vi "Command Buffer.vi"(2 "All Robot Commands In":T1, 3 "Startup":bool, 4 "String Parameter":string, 5 "Cmd Parameter 3":dbl, 6 "Cmd Parameter 2":dbl, 7 "Cmd Parameter 1":dbl) -> (0 "All Robot Commands Out":T1, 1 "Completed":bool)   [LabVIEW 2016]
uses:
  Subsystems/All Robot Commands.ctl
  Subsystems/Drive and Climb SS/Drive + Climb Commands 2017.ctl
  Subsystems/Gear Delivery SS/Gear Delivery Commands.ctl
  Subsystems/Conveyor and Shooter SS/Conveyor and Shooter Commands.ctl
  Subsystems/Ball Intake SS/Ball Intake Commands.ctl
  Command Execution State.ctl
  Global Variables/Folder Names.vi
  Global Variables/MotionProfile.vi
  <vilib>/Utility/file.llb/Read Delimited Spreadsheet (DBL).vi
  Global Variables/Refnum Names.vi
panel:
  out "Total Points in File":i32
  # "Sample robot\ncontrol output.\nReplace with \nactual teleop \ncontrol signal \nstructure."
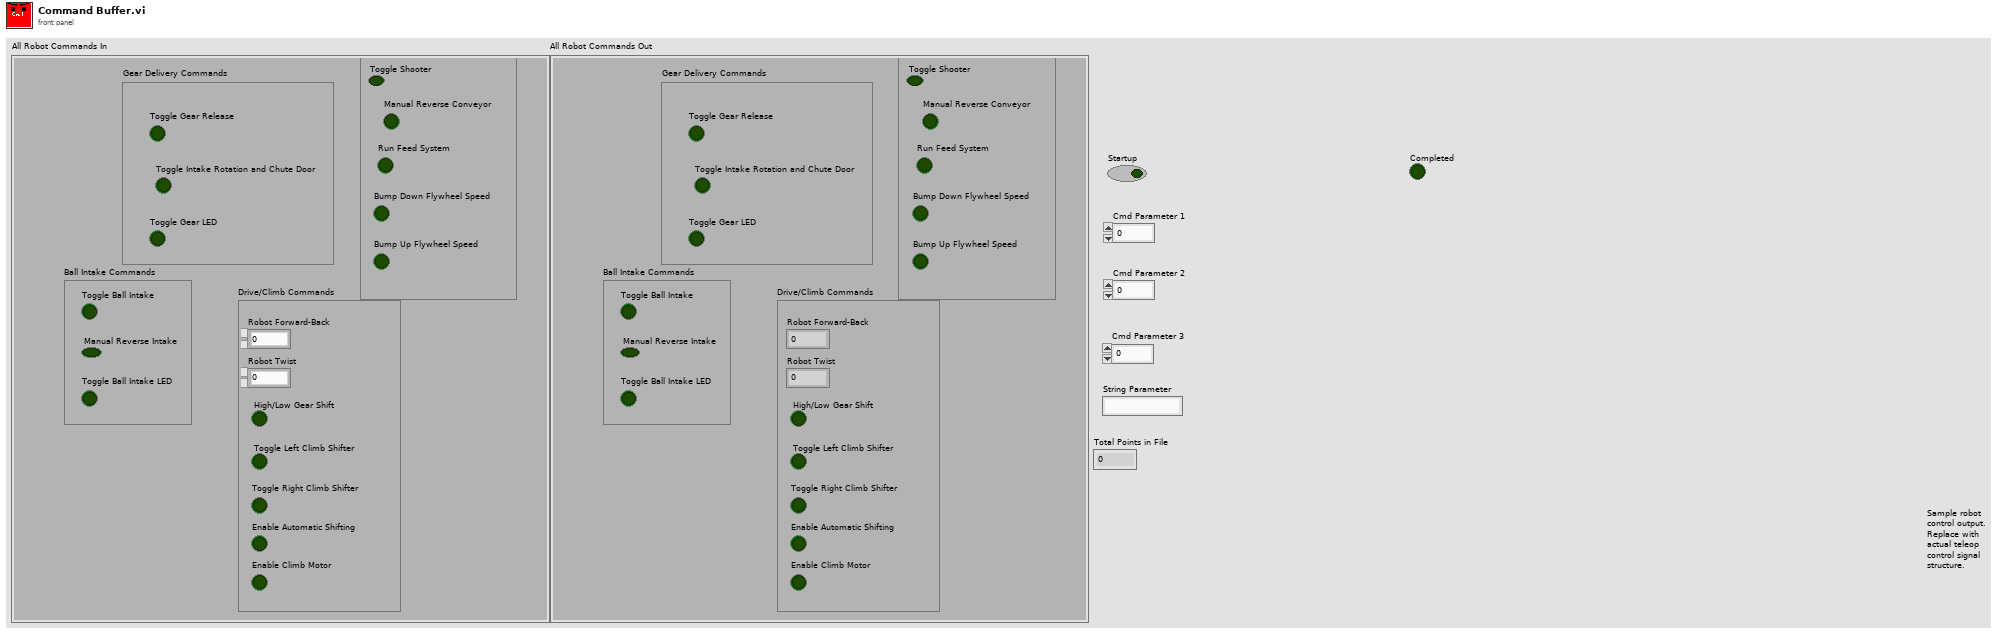
[diagram p1: front panel]
types:
  T1 = typedef "All Robot Commands.ctl" = cluster{"Drive/Climb Commands":T2, "Gear Delivery Commands":T3, "Shooter and Conveyor Commands":T4, "Ball Intake Commands":T5}
  T2 = typedef "Drive + Climb Commands 2017.ctl" = cluster{"Robot Forward-Back":dbl, "Robot Twist":dbl, "High/Low Gear Shift":bool, "Toggle Left Climb Shifter":bool, "Toggle Right Climb Shifter":bool, "Enable Automatic Shifting":bool, "Enable Climb Motor ":bool}
  T3 = typedef "Gear Delivery Commands.ctl" = cluster{"Toggle Gear Release":bool, "Toggle Intake Rotation and Chute Door":bool, "Toggle Gear LED":bool}
  T4 = typedef "Conveyor and Shooter Commands.ctl" = cluster{"Toggle Shooter":bool, "Manual Reverse Conveyor":bool, "Run Feed System":bool, "Bump Down Flywheel Speed":bool, "Bump Up Flywheel Speed":bool}
  T5 = typedef "Ball Intake Commands.ctl" = cluster{"Toggle Ball Intake":bool, "Manual Reverse Intake":bool, "Toggle Ball Intake LED":bool}
  T6 = typedef "Command Execution State.ctl" = enum16{"Initialize", "Execute", "Finish"}
  T7 = typedef "MotionProfile TypeDef.ctl" = cluster{"Left MP Array":dbl[][], "Left MP Index":dbl, "Semaphore":bool, "Right MP Array":dbl[][], "Right MP Index":dbl}
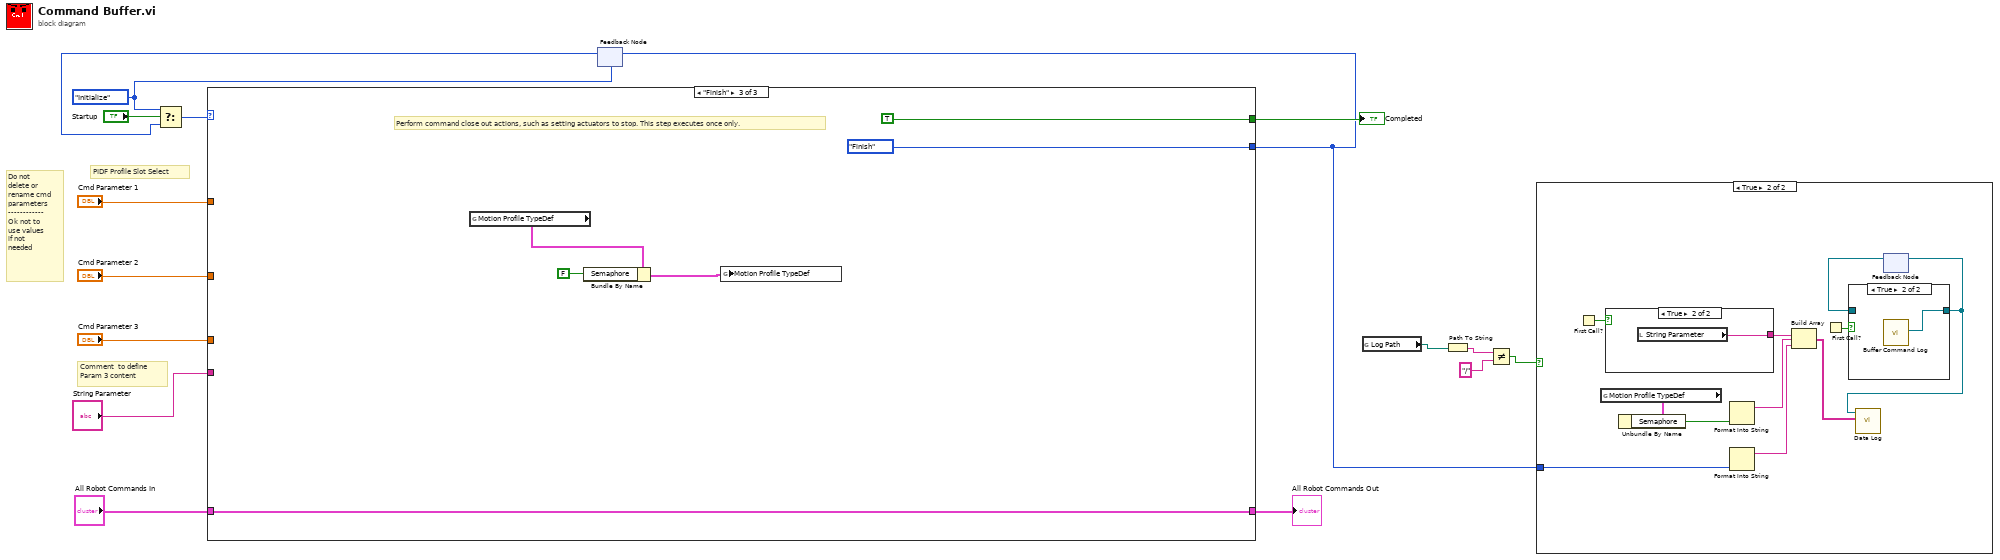
[diagram p0: block diagram]
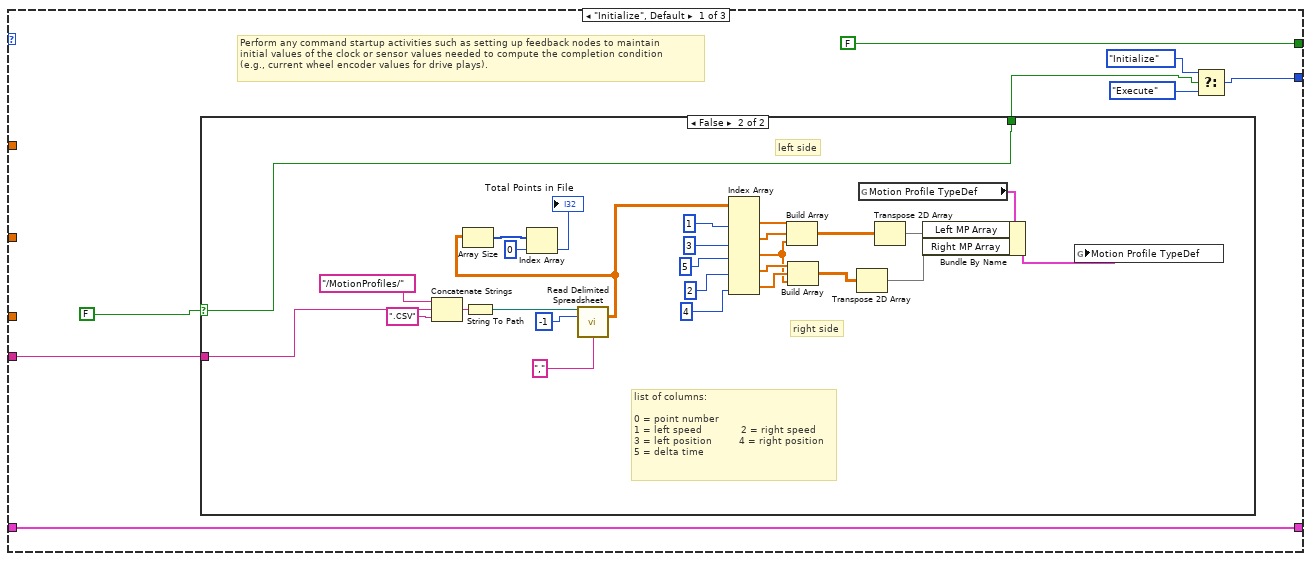
[diagram p5: hidden frame]
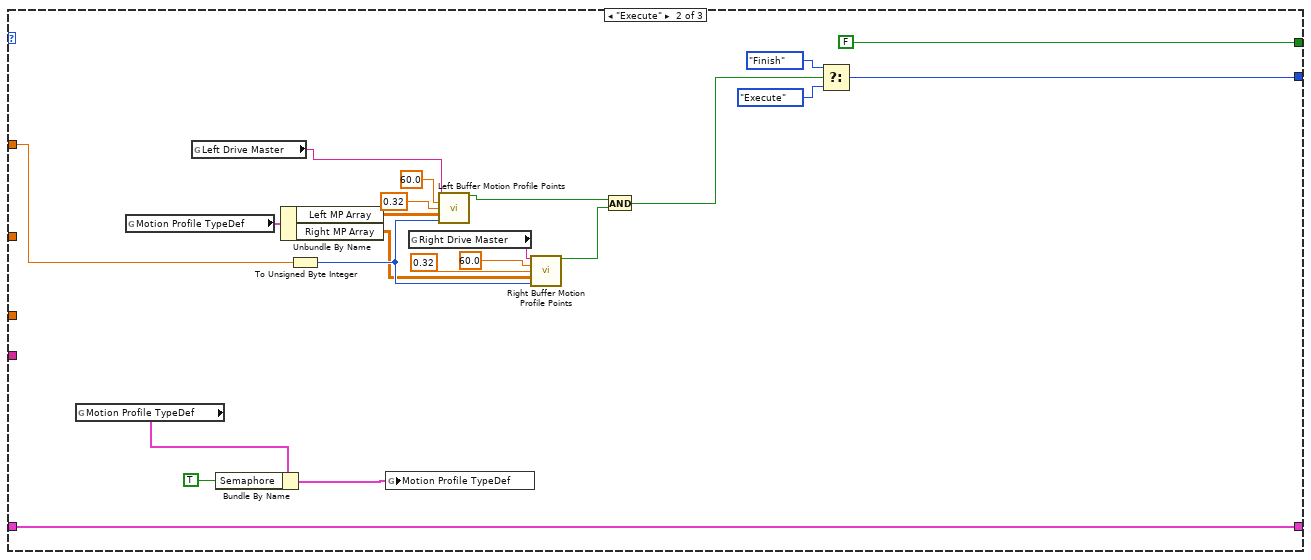
[diagram p7: hidden frame]
diagram:
  w12 = Command_Execution_State."Initialize" ("Play State")
  # "Comment  to define\nParam 3 content"
  # "PIDF Profile Slot Select"
  # "Do not \ndelete or\nrename cmd\nparameters\n------------\nOk not to \nuse values\nif not \nneeded"
  n1 = feedback #1(w12) -> (w13:T6)
  n2 = Select(t=w12, s="Startup", f=w13) -> (s? t:f=w16:T6)
  n3 = case shown="\"Finish\"" w16 {
    tunnel: [FALSE FALSE TRUE] -> w14
    tunnel: [w22 w73 Command_Execution_State."Finish" ("f")] -> w5
    tunnel: "Cmd Parameter 1" -> [_ w68 _]
    tunnel: "Cmd Parameter 2" -> [_ _ _]
    tunnel: "Cmd Parameter 3" -> [_ _ _]
    tunnel: "String Parameter" -> [w23 _ _]
    tunnel: "All Robot Commands In" -> [w18 w54 w76]
    tunnel: [w18 w54 w76] -> w6
    frame "Initialize", Default {
      # "Perform any command startup activities such as setting up feedback nodes to maintain \ninitial values of the clock or sensor values needed to compute the completion condition\n(e.g., current wheel encoder values for drive plays)."
      n4 = case shown="False" FALSE {
        selector: FALSE -> [w25 w27]
        tunnel: w23 -> [_ w50]
        tunnel: [w25 w27] -> w19
        frame True {
        }
        frame False {
          # "list of columns:\n\n0 = point number\n1 = left speed             2 = right speed\n3 = left position         4 = right position\n5 = delta time"
          # "left side"
          # "right side"
          n5 = Concatenate Strings("/MotionProfiles/" ("string"), w50, ".CSV" ("string")) -> (w51:string)
          n6 = String To Path(string=w51) -> (path=w26:path)
          n7 = call-poly <vilib>:"Read Delimited Spreadsheet.vi"("file path (dialog if empty)"=w26, "number of rows (all:-1)"=-1, "delimiter (\\t)"="," ("delimiter (\\t)")) -> ("all rows"=w34:dbl[][])  [unwired: 7 in, 5 out]
          n8 = Array Size(array=w34) -> (size(s)=w33:i32[])
          n9 = Index Array(array=w33, index=0) -> (element=→"Total Points in File":i32)
          n10 = Index Array(array=w34, index (col) #1=1 ("disabled index (col)"), index (col) #2=3 ("disabled index (col)"), index (col) #3=5 ("disabled index (col)"), index (col) #4=2 ("disabled index (col)"), index (col) #5=4 ("disabled index (col)")) -> (element #1=w41:dbl[], element #2=w40:dbl[], element #3=w37:dbl[], element #4=w39:dbl[], element #5=w38:dbl[])  [unwired: 5 in]
          n11 = Build Array(w41, w40, w37) -> (w36:dbl[][])
          n12 = Build Array(w39, w38, w37) -> (w35:dbl[][])
          n13 = Transpose 2D Array(2D array=w35) -> (transposed array=w28:dbl[][])
          n14 = global read "MotionProfile.vi" "Motion Profile TypeDef"() -> (w30:T7)
          n15 = Transpose 2D Array(2D array=w36) -> (transposed array=w29:dbl[][])
          n16 = Bundle By Name(cluster=w30, "Left MP Array"=w29, "Right MP Array"=w28) -> (w31:T7)
          n17 = global write "MotionProfile.vi" "Motion Profile TypeDef"(w31) -> ()
        }
      }
      n18 = Select(t=Command_Execution_State."Initialize" ("Play State"), s=w19, f=Command_Execution_State."Execute" ("Play State")) -> (s? t:f=w22:T6)
    }
    frame "Execute" {
      n19 = global read "MotionProfile.vi" "Motion Profile TypeDef"() -> (w59:T7)
      n20 = global read "MotionProfile.vi" "Motion Profile TypeDef"() -> (w71:T7)
      n21 = global read "Refnum Names.vi" "Left Drive Master"() -> (w56:string)
      n22 = Bundle By Name(cluster=w59, "Semaphore"=TRUE) -> (w57:T7)
      n23 = Unbundle By Name(w71) -> ("Left MP Array"=w70:dbl[][], "Right MP Array"=w63:dbl[][])
      n24 = To Unsigned Byte Integer(number=w68) -> (unsigned 8bit integer=w69:u8)
      n25 = global write "MotionProfile.vi" "Motion Profile TypeDef"(w57) -> ()
      n26 = global read "Refnum Names.vi" "Right Drive Master"() -> (w55:string)
      n27 = call "Left Buffer Motion Profile Points.vi"("Motor Name"=w56, "Time Conversion Factor"=60.0, "Linear Conversion Factor"=0.32, "Motion Profile Array"=w70, "PIDF Profile Slot Select"=w69) -> ("Ready to Execute"=w62:bool)  [unwired: 10 in]
      n28 = call "Right Buffer Motion Profile Points.vi"("Motor Name"=w55, "Time Conversion Factor"=60.0, "Linear Conversion Factor"=0.32, "Motion Profile Array"=w63, "PIDF Profile Slot Select"=w69) -> ("Ready to Execute"=w61:bool)  [unwired: 10 in]
      n29 = And(x=w62, y=w61) -> (x .and. y?=w60:bool)
      n30 = Select(t=Command_Execution_State."Finish" ("Play State"), s=w60, f=Command_Execution_State."Execute") -> (s? t:f=w73:T6)
    }
    frame "Finish" {
      # "Perform command close out actions, such as setting actuators to stop. This step executes once only."
      n31 = global read "MotionProfile.vi" "Motion Profile TypeDef"() -> (w79:T7)
      n32 = Bundle By Name(cluster=w79, "Semaphore"=FALSE) -> (w77:T7)
      n33 = global write "MotionProfile.vi" "Motion Profile TypeDef"(w77) -> ()
    }
  }
  "Completed" <- w14
  "All Robot Commands Out" <- w6
  n34 = feedback-in #1(w5) -> ()
  n35 = global read "Folder Names.vi" "Log Path"() -> (w4:path)
  n36 = Path To String(path=w4) -> (string=w3:string)
  n37 = Not Equal?(x=w3, y="/") -> (x != y?=w1:bool)
  n38 = case shown="True" w1 {
    tunnel: w5 -> [_ w83]
    frame False {
    }
    frame True {
      n39 = First Call?() -> (First Call?: T/F=w89:bool)
      n40 = global read "MotionProfile.vi" "Motion Profile TypeDef"() -> (w87:T7)
      n41 = case shown="True" w89 {
        tunnel: [_ w93] -> w86
        frame False {
        }
        frame True {
          n42 = local read "String Parameter"() -> (w93:string)
        }
      }
      n43 = Unbundle By Name(w87) -> ("Semaphore"=w88:bool)
      n44 = Format Into String(w88) -> (resulting string=w85:string)  [unwired: 3 in, 1 out]
      n45 = Format Into String(w83) -> (resulting string=w82:string)  [unwired: 3 in, 1 out]
      n46 = Build Array(w86, w85, w82) -> (w84:string[])
      n47 = First Call?() -> (First Call?: T/F=w92:bool)
      n48 = feedback #2() -> (w91:refnum<file>)  [unwired: 1 in]
      n49 = case shown="True" w92 {
        tunnel: [w94 w95] -> w90
        tunnel: w91 -> [w94 _]
        frame False {
        }
        frame True {
          n50 = call "Buffer Command Log.vi"() -> ("File Reference Out"=w95:refnum<file>)  [unwired: 11 in]
        }
      }
      n51 = call "Data Log.vi"("Data In"=w84, "File Reference In"=w90) -> ()  [unwired: 9 in, 1 out]
      n52 = feedback-in #2(w90) -> ()
    }
  }
